vi "ApplyJitter.vi"(0 "ValueIn":dbl, 1 "JitterFraction":dbl=0.2) -> (2 "JitteredValueOut":dbl)   [LabVIEW 2011]
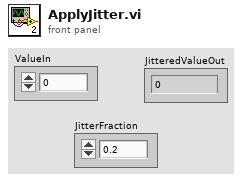
[diagram p1: front panel]
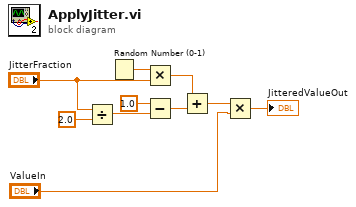
[diagram p0: block diagram]
diagram:
  n1 = Divide(x="JitterFraction", y=2.0) -> (x/y=w2:dbl)
  n2 = Random Number (0-1)() -> (number: 0 to 1=w4:dbl)
  n3 = Multiply(x=w4, y="JitterFraction") -> (x*y=w3:dbl)
  n4 = Subtract(x=1.0, y=w2) -> (x-y=w5:dbl)
  n5 = Add(x=w3, y=w5) -> (x+y=w8:dbl)
  n6 = Multiply(x=w8, y="ValueIn") -> (x*y=→"JitteredValueOut":dbl)
